vi "InitializeAsGRPC.vi"(8 "error in (no error)":errorcluster, 10 "MicronConfig":T1, 11 "Service":T2) -> (0 "error out":errorcluster, 2 "MessageUserEvent":refnum<user-event>, 3 "MicronServer":refnum<class "ServiceBase.lvclass">)   [LabVIEW 2019, in "MicronGRPCServer.lvlib" / "GRPCService.lvclass"]
uses:
  GRPCService.lvclass
  Base/Server/Message/MessageBase.lvclass
  Base/Server/Service/ServiceBase.lvclass
  Base/Server/Service/Typedefs/MicronArgs.ctl
  D:/GitHub/KarthikAbiram/Micron/LabVIEW/Source/vi.lib/Micron/Base/Server/Service/ServiceBase.lvclass
  Base/Server/Service/Typedefs/MicronConfig.ctl
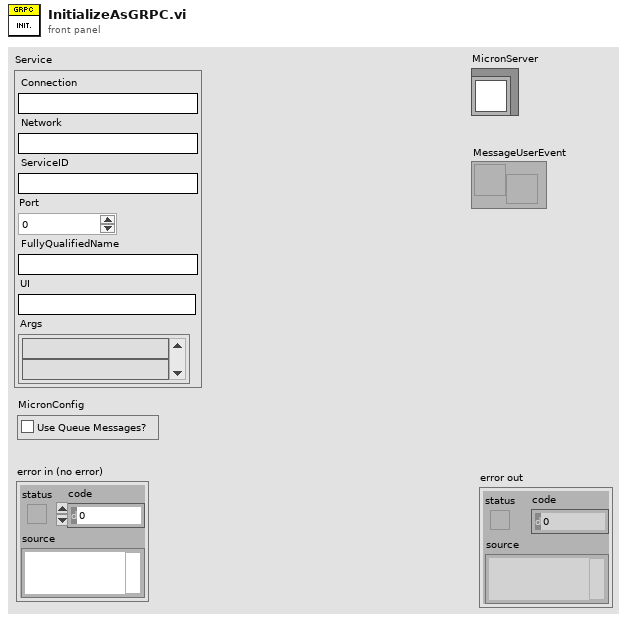
[diagram p1: front panel]
types:
  T1 = typedef "MicronServer.lvlib/ServiceBase.lvclass/MicronConfig.ctl" = cluster{"Use Queue Messages?":bool}
  T2 = typedef "MicronServer.lvlib/ServiceBase.lvclass/MicronArgs.ctl" = cluster{"Connection":string, "Network":string, "ServiceID":string, "Port":i32, "FullyQualifiedName":string, "UI":string, "Args":string[]}
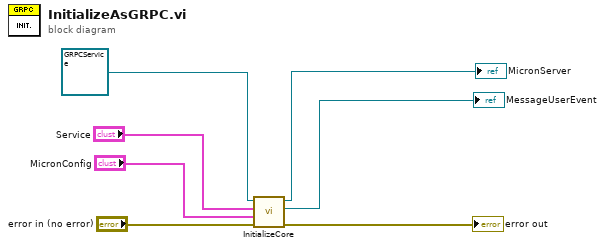
[diagram p0: block diagram]
diagram:
  n1 = call-dynamic "InitializeCore.vi"("error in (no error)"="error in (no error)", "MicronConfig"="MicronConfig", "Micron Args"="Service", "MicronServer in"=refnum<class "GRPCService.lvclass"> refnum) -> ("error out"=→"error out":errorcluster, "MessageUserEvent"=→"MessageUserEvent":refnum<user-event>, "MicronServer out"=→"MicronServer":refnum<class "GRPCService.lvclass">)  [unwired: 5 in]
